vi "New JSON Boolean.vi"(8 "error in (no error)":errorcluster, 10 "value":bool) -> (0 "error out":errorcluster, 3 "JSON String out":refnum<class "JSON Boolean.lvclass">)   [LabVIEW 2015, in "LVJSON.lvlib" / "JSON Boolean.lvclass"]
uses:
  JSON Boolean.lvclass
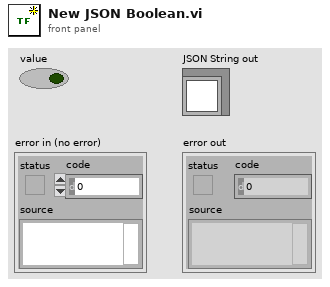
[diagram p1: front panel]
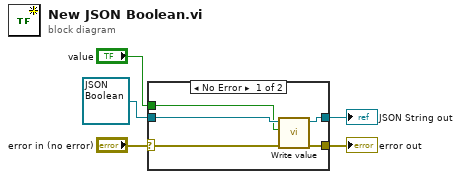
[diagram p0: block diagram]
diagram:
  n1 = case shown="No Error" "error in (no error)" {
    selector: "error in (no error)" -> [w7 w12]
    tunnel: [w9 w12] -> w4
    tunnel: [w10 w11] -> w2
    tunnel: refnum<class "JSON Boolean.lvclass"> refnum ("JSON String in") -> [w8 w11]
    tunnel: "value" -> [w6 _]
    frame No Error {
      n2 = call-dynamic "Write value.vi"("error in (no error)"=w7, "value"=w6, "JSON String in"=w8) -> ("error out"=w9:errorcluster, "JSON String out"=w10:refnum<class "JSON Boolean.lvclass">)  [unwired: 7 in]
    }
    frame Error {
    }
  }
  "error out" <- w4
  "JSON String out" <- w2
